vi "LibXML_CloseFile.vi"(8 "error in":errorcluster, 11 "doc":u32) -> (0 "error out":errorcluster)   [LabVIEW 2019, in "Tools.lvlib" / "LibXML.lvlib"]
doc: "Close a file or document opened as a string. Input doc handle. Should be used for all docs."
uses:
  LibXML.lvlib
  dll/libxml2.dll
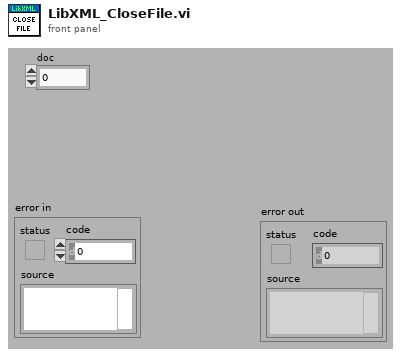
[diagram p1: front panel]
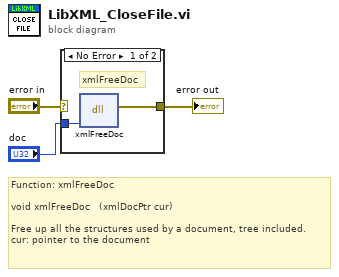
[diagram p0: block diagram]
diagram:
  # "Function: xmlFreeDoc\n\nvoid\txmlFreeDoc\t\t\t(xmlDocPtr cur)\n\nFree up all the structures used by a document, tree included.\ncur:\tpointer to the document"
  n1 = case shown="No Error" "error in" {
    selector: "error in" -> [_ w6]
    tunnel: [w5 w6] -> w2
    tunnel: "doc" -> [w4 _]
    frame No Error {
      # "xmlFreeDoc"
      n2 = dll-call lib="C:/Projects/_Prywatne/MyCIT/Framework/Tools/XML/LibXML/dll/libxml2.dll" fn="xmlFreeDoc"("doc"=w4) -> (error out=w5:errorcluster)  [unwired: 5 in, 1 out]
    }
    frame Error {
    }
  }
  "error out" <- w2
